vi "ADCP_UI_Queue_Manager.vi"(8 "error in (no error)":errorcluster, 10 "command":T1, 11 "ADCU_GUI References":T2) -> (0 "error out":errorcluster)   [LabVIEW 2017]
uses:
  Controls/ADCP_UI/ADCP_UI_Parameters.ctl
  Controls/ADCP_UI/ADCP_UI_Queues.ctl
  Controls/ADCP_UI/ADCP_UI_Continuous_Receiver_States.ctl
  Controls/ADCP_UI/ADCP_Queue_Receive_Log_Queue_Element.ctl
  Controls/Packet/Packet.ctl
  Controls/Packet/Packet_Direction.ctl
  Controls/Packet/Packet_Type.ctl
  Controls/Packet/Packet_Priority.ctl
  Controls/Data Packets/Data_Packet.ctl
  Controls/Data Packets/Parameter.ctl
  Controls/Data Packets/Parameter_Data_Type.ctl
  Controls/Data Packets/Data_Packet_Transmit_Mode.ctl
  Controls/ADCP_UI/ADCP_UI_Queue_Manager_Commands.ctl
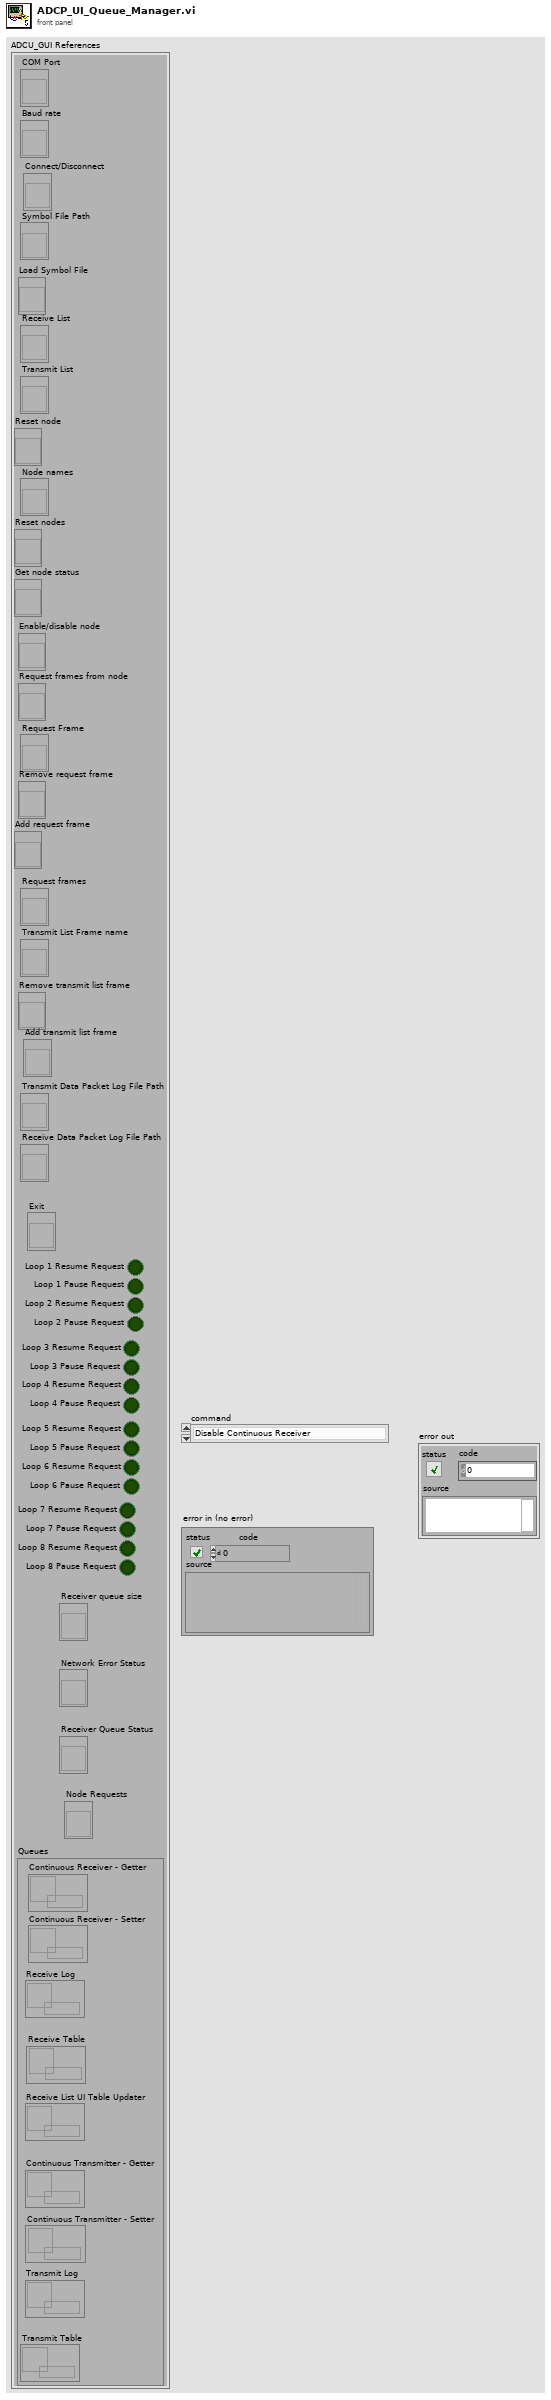
[diagram p1: front panel]
types:
  T1 = typedef "ADCP_UI_Queue_Manager_Commands.ctl" = enum16{"Disable Continuous Receiver", "Enable Continuous Receiver", "Disable Continuous Transmitter", "Enable Continuous Transmitter", "Enable Continuous Tx & Rx", "Disable Continuous Tx & Rx"}
  T2 = typedef "ADCP_UI_Parameters.ctl" = cluster{"COM Port":refnum<vi>, "Baud rate":refnum<vi>, "Symbol File Path":refnum<vi>, "Receive List":refnum<vi>, "Transmit List":refnum<vi>, "Node names":refnum<vi>, "Request Frame":refnum<vi>, "Request frames":refnum<vi>, "Transmit List Frame name":refnum<vi>, "Transmit Data Packet Log File Path":refnum<vi>, "Receive Data Packet Log File Path":refnum<vi>, "Loop 1 Resume Request":bool, "Loop 1 Pause Request":bool, "Loop 2 Resume Request":bool, "Loop 2 Pause Request":bool, "Loop 3 Resume Request":bool, "Loop 3 Pause Request":bool, "Loop 4 Resume Request":bool, "Loop 4 Pause Request":bool, "Loop 5 Resume Request":bool, "Loop 5 Pause Request":bool, "Loop 6 Resume Request":bool, "Loop 6 Pause Request":bool, "Loop 7 Resume Request":bool, "Loop 7 Pause Request":bool, "Loop 8 Resume Request":bool, "Loop 8 Pause Request":bool, "Exit":refnum<vi>, "Connect/Disconnect":refnum<vi>, "Load Symbol File":refnum<vi>, "Reset node":refnum<vi>, "Reset nodes":refnum<vi>, "Get node status":refnum<vi>, "Enable/disable node":refnum<vi>, "Request frames from node":refnum<vi>, "Remove request frame":refnum<vi>, "Add request frame":refnum<vi>, "Remove transmit list frame":refnum<vi>, "Add transmit list frame":refnum<vi>, "Receiver queue size":refnum<vi>, "Network Error Status":refnum<vi>, "Receiver Queue Status":refnum<vi>, "Node Requests":refnum<vi>, "Queues":T3}
  T3 = typedef "ADCP_UI_Queues.ctl" = cluster{"Continuous Receiver - Getter":refnum<queue>, "Continuous Receiver - Setter":refnum<queue>, "Receive Log":refnum<queue>, "Receive Table":refnum<queue>, "Receive List UI Table Updater":refnum<queue>, "Continuous Transmitter - Getter":refnum<queue>, "Continuous Transmitter - Setter":refnum<queue>, "Transmit Log":refnum<queue>, "Transmit Table":refnum<queue>}
  T4 = typedef "ADCP_UI_Continuous_Receiver_States.ctl" = enum16{"Disable", "Enable", "Exit"}
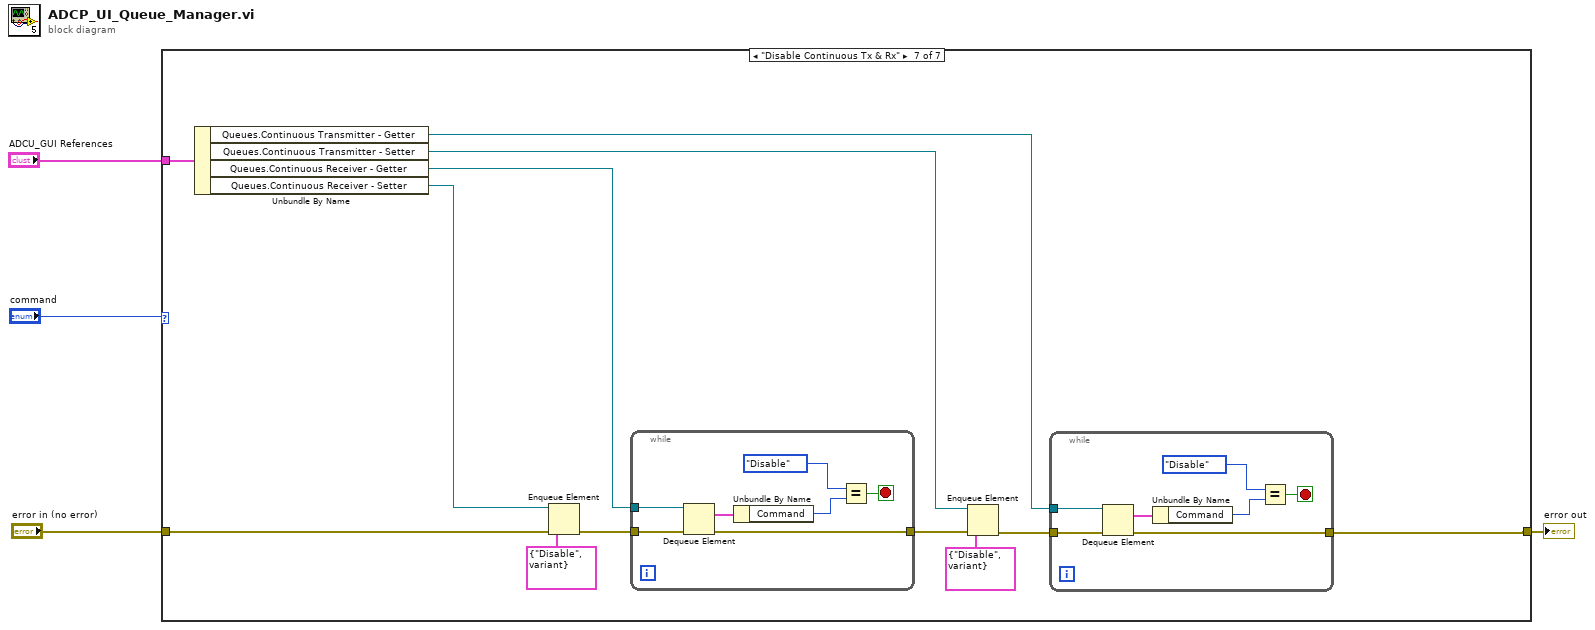
[diagram p0: block diagram]
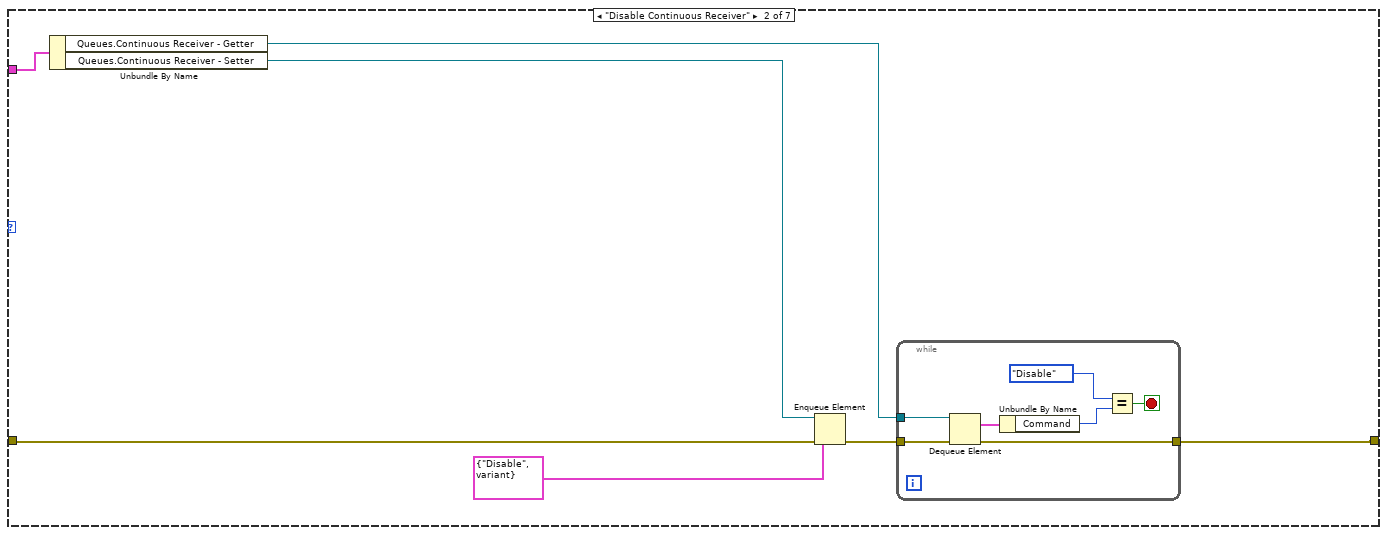
[diagram p3: hidden frame]
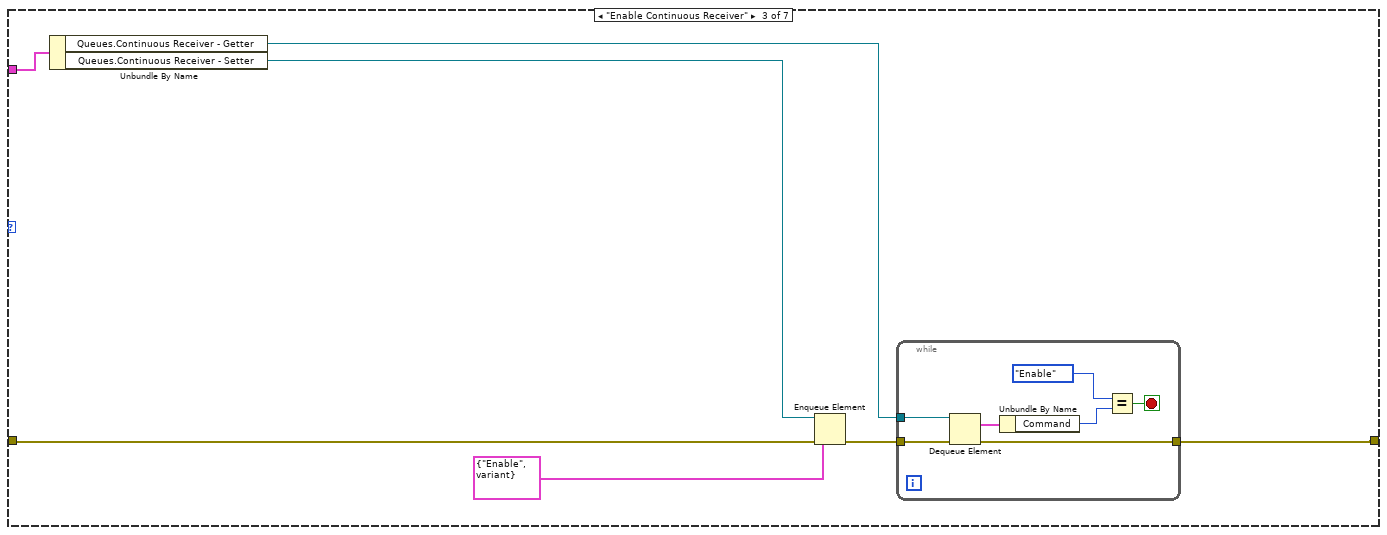
[diagram p4: hidden frame]
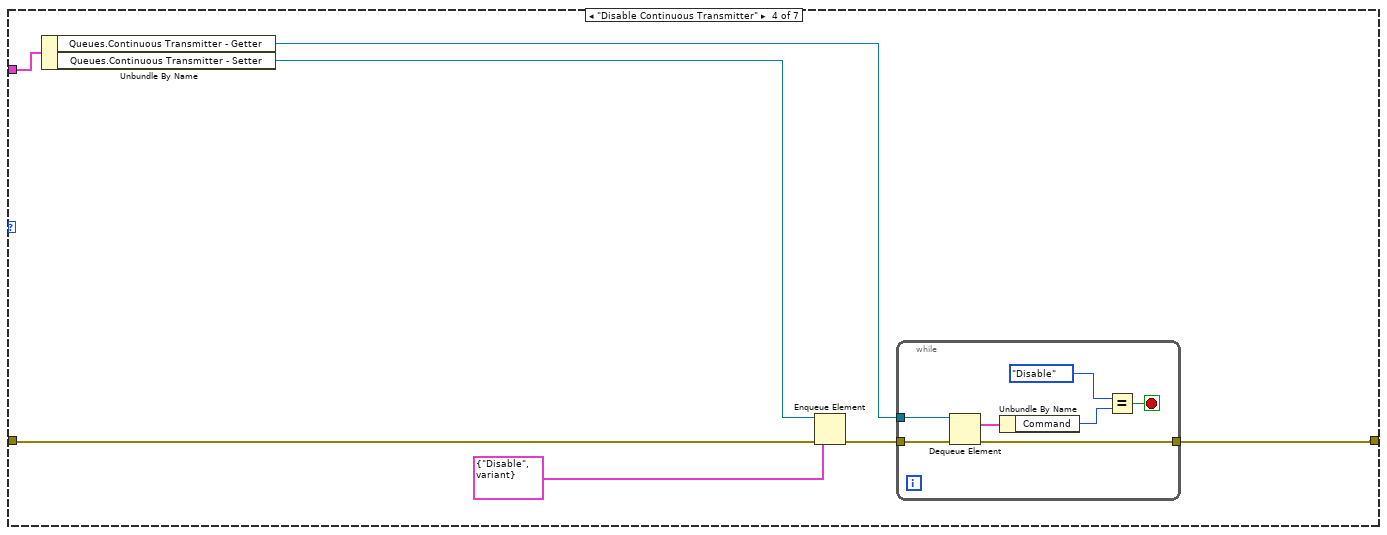
[diagram p5: hidden frame]
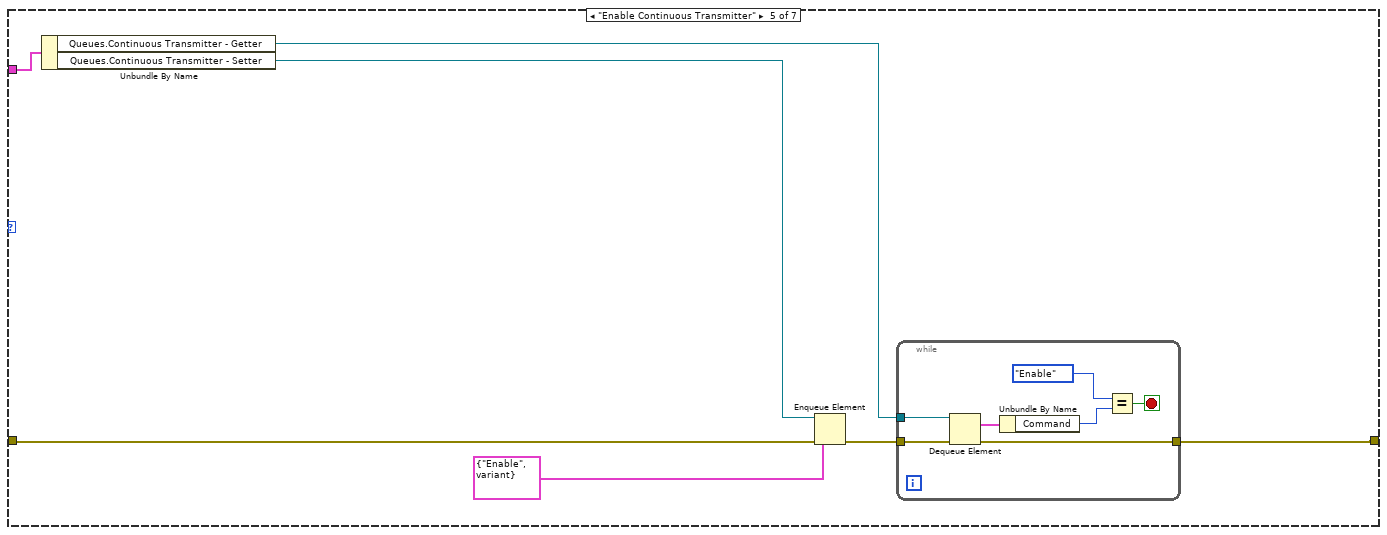
[diagram p6: hidden frame]
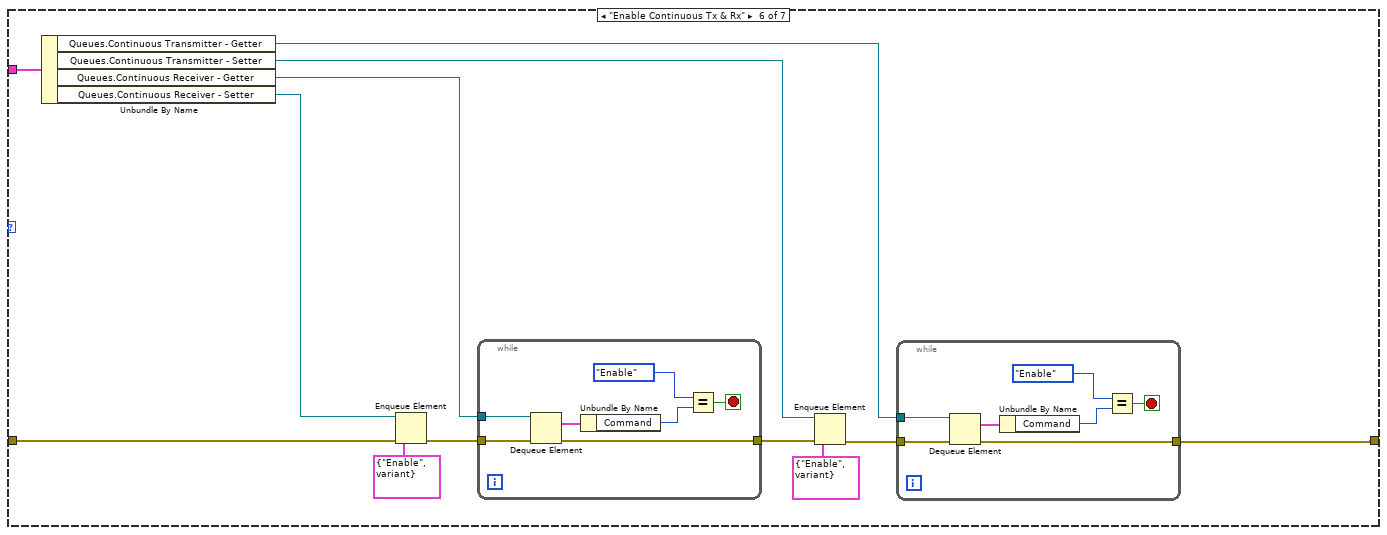
[diagram p7: hidden frame]
diagram:
  n1 = case shown="\"Disable Continuous Tx & Rx\"" "command" {
    tunnel: "error in (no error)" -> [w5 w11 w25 w39 w53 w65 w91]
    tunnel: [w5 w6 w20 w34 w48 w68 w94] -> w1
    tunnel: "ADCU_GUI References" -> [_ w12 w26 w40 w54 w73 w99]
    frame Default {
    }
    frame "Disable Continuous Receiver" {
      n2 = Unbundle By Name(w12) -> ("Queues.Continuous Receiver - Getter"=w7:refnum<queue>, "Queues.Continuous Receiver - Setter"=w10:refnum<queue>)
      n3 = Enqueue Element(queue=w10, element=cluster{"Command":T4, "Data":variant} {"Command"=enum."Disable", "Data"=variant}, error in (no error)=w11) -> (error out=w8:errorcluster)  [unwired: 1 in, 2 out]
      n4 = while {
        tunnel: w8 -> [w19]
        tunnel: w7 -> [w18]
        tunnel: [w13] -> w6
        stop <- w14 stop-if-true
        n5 = Dequeue Element(queue=w18, error in (no error)=w19) -> (element=w17:cluster{"Command":T4, "Data":variant}, error out=w13:errorcluster)  [unwired: 1 in, 2 out]
        n6 = Unbundle By Name(w17) -> ("Command"=w16:T4)
        n7 = Equal?(x=ADCP_UI_Continuous_Receiver_States."Disable", y=w16) -> (x = y?=w14:bool)
      }
    }
    frame "Enable Continuous Receiver" {
      n8 = Unbundle By Name(w26) -> ("Queues.Continuous Receiver - Getter"=w21:refnum<queue>, "Queues.Continuous Receiver - Setter"=w24:refnum<queue>)
      n9 = Enqueue Element(queue=w24, element=cluster{"Command":T4, "Data":variant} {"Command"=enum."Enable", "Data"=variant}, error in (no error)=w25) -> (error out=w22:errorcluster)  [unwired: 1 in, 2 out]
      n10 = while {
        tunnel: w22 -> [w33]
        tunnel: w21 -> [w32]
        tunnel: [w27] -> w20
        stop <- w28 stop-if-true
        n11 = Dequeue Element(queue=w32, error in (no error)=w33) -> (element=w31:cluster{"Command":T4, "Data":variant}, error out=w27:errorcluster)  [unwired: 1 in, 2 out]
        n12 = Unbundle By Name(w31) -> ("Command"=w30:T4)
        n13 = Equal?(x=ADCP_UI_Continuous_Receiver_States."Enable", y=w30) -> (x = y?=w28:bool)
      }
    }
    frame "Disable Continuous Transmitter" {
      n14 = Unbundle By Name(w40) -> ("Queues.Continuous Transmitter - Getter"=w35:refnum<queue>, "Queues.Continuous Transmitter - Setter"=w38:refnum<queue>)
      n15 = Enqueue Element(queue=w38, element=cluster{"Command":T4, "Data":variant} {"Command"=enum."Disable", "Data"=variant}, error in (no error)=w39) -> (error out=w36:errorcluster)  [unwired: 1 in, 2 out]
      n16 = while {
        tunnel: w36 -> [w47]
        tunnel: w35 -> [w46]
        tunnel: [w41] -> w34
        stop <- w42 stop-if-true
        n17 = Dequeue Element(queue=w46, error in (no error)=w47) -> (element=w45:cluster{"Command":T4, "Data":variant}, error out=w41:errorcluster)  [unwired: 1 in, 2 out]
        n18 = Unbundle By Name(w45) -> ("Command"=w44:T4)
        n19 = Equal?(x=ADCP_UI_Continuous_Receiver_States."Disable", y=w44) -> (x = y?=w42:bool)
      }
    }
    frame "Enable Continuous Transmitter" {
      n20 = Unbundle By Name(w54) -> ("Queues.Continuous Transmitter - Getter"=w49:refnum<queue>, "Queues.Continuous Transmitter - Setter"=w52:refnum<queue>)
      n21 = Enqueue Element(queue=w52, element=cluster{"Command":T4, "Data":variant} {"Command"=enum."Enable", "Data"=variant}, error in (no error)=w53) -> (error out=w50:errorcluster)  [unwired: 1 in, 2 out]
      n22 = while {
        tunnel: w50 -> [w61]
        tunnel: w49 -> [w60]
        tunnel: [w55] -> w48
        stop <- w56 stop-if-true
        n23 = Dequeue Element(queue=w60, error in (no error)=w61) -> (element=w59:cluster{"Command":T4, "Data":variant}, error out=w55:errorcluster)  [unwired: 1 in, 2 out]
        n24 = Unbundle By Name(w59) -> ("Command"=w58:T4)
        n25 = Equal?(x=ADCP_UI_Continuous_Receiver_States."Enable", y=w58) -> (x = y?=w56:bool)
      }
    }
    frame "Enable Continuous Tx & Rx" {
      n26 = Unbundle By Name(w73) -> ("Queues.Continuous Transmitter - Getter"=w69:refnum<queue>, "Queues.Continuous Transmitter - Setter"=w72:refnum<queue>, "Queues.Continuous Receiver - Getter"=w63:refnum<queue>, "Queues.Continuous Receiver - Setter"=w64:refnum<queue>)
      n27 = Enqueue Element(queue=w64, element=cluster{"Command":T4, "Data":variant} {"Command"=enum."Enable", "Data"=variant}, error in (no error)=w65) -> (error out=w66:errorcluster)  [unwired: 1 in, 2 out]
      n28 = while {
        tunnel: w66 -> [w80]
        tunnel: w63 -> [w79]
        tunnel: [w74] -> w62
        stop <- w75 stop-if-true
        n29 = Dequeue Element(queue=w79, error in (no error)=w80) -> (element=w78:cluster{"Command":T4, "Data":variant}, error out=w74:errorcluster)  [unwired: 1 in, 2 out]
        n30 = Unbundle By Name(w78) -> ("Command"=w77:T4)
        n31 = Equal?(x=ADCP_UI_Continuous_Receiver_States."Enable", y=w77) -> (x = y?=w75:bool)
      }
      n32 = Enqueue Element(queue=w72, element=cluster{"Command":T4, "Data":variant} {"Command"=enum."Enable", "Data"=variant}, error in (no error)=w62) -> (error out=w70:errorcluster)  [unwired: 1 in, 2 out]
      n33 = while {
        tunnel: w70 -> [w87]
        tunnel: w69 -> [w86]
        tunnel: [w81] -> w68
        stop <- w82 stop-if-true
        n34 = Dequeue Element(queue=w86, error in (no error)=w87) -> (element=w85:cluster{"Command":T4, "Data":variant}, error out=w81:errorcluster)  [unwired: 1 in, 2 out]
        n35 = Unbundle By Name(w85) -> ("Command"=w84:T4)
        n36 = Equal?(x=ADCP_UI_Continuous_Receiver_States."Enable", y=w84) -> (x = y?=w82:bool)
      }
    }
    frame "Disable Continuous Tx & Rx" {
      n37 = Unbundle By Name(w99) -> ("Queues.Continuous Transmitter - Getter"=w95:refnum<queue>, "Queues.Continuous Transmitter - Setter"=w98:refnum<queue>, "Queues.Continuous Receiver - Getter"=w89:refnum<queue>, "Queues.Continuous Receiver - Setter"=w90:refnum<queue>)
      n38 = Enqueue Element(queue=w90, element=cluster{"Command":T4, "Data":variant} {"Command"=enum."Disable", "Data"=variant}, error in (no error)=w91) -> (error out=w92:errorcluster)  [unwired: 1 in, 2 out]
      n39 = while {
        tunnel: w92 -> [w106]
        tunnel: w89 -> [w105]
        tunnel: [w100] -> w88
        stop <- w101 stop-if-true
        n40 = Dequeue Element(queue=w105, error in (no error)=w106) -> (element=w104:cluster{"Command":T4, "Data":variant}, error out=w100:errorcluster)  [unwired: 1 in, 2 out]
        n41 = Unbundle By Name(w104) -> ("Command"=w103:T4)
        n42 = Equal?(x=ADCP_UI_Continuous_Receiver_States."Disable", y=w103) -> (x = y?=w101:bool)
      }
      n43 = Enqueue Element(queue=w98, element=cluster{"Command":T4, "Data":variant} {"Command"=enum."Disable", "Data"=variant}, error in (no error)=w88) -> (error out=w96:errorcluster)  [unwired: 1 in, 2 out]
      n44 = while {
        tunnel: w96 -> [w113]
        tunnel: w95 -> [w112]
        tunnel: [w107] -> w94
        stop <- w108 stop-if-true
        n45 = Dequeue Element(queue=w112, error in (no error)=w113) -> (element=w111:cluster{"Command":T4, "Data":variant}, error out=w107:errorcluster)  [unwired: 1 in, 2 out]
        n46 = Unbundle By Name(w111) -> ("Command"=w110:T4)
        n47 = Equal?(x=ADCP_UI_Continuous_Receiver_States."Disable", y=w110) -> (x = y?=w108:bool)
      }
    }
  }
  "error out" <- w1
